vi "CRYHardware Global.vi"() -> ()   [LabVIEW 2013]
panel:
  out "Mic Vol-R backup":dbl
  out "Mic Vol-L backup":dbl
  out "Input Channel 1/2 Index backup":i32
  out "Impedance 1 index backup":i32
  out "Mic Voltage backup":dbl
  out "Mic Res-R backup":dbl
  out "Mic Res-L backup":dbl
  out "Mic Resister backup":dbl
  out "Impedance 2  backup":i32
  out "Impedance 1  backup":i32
  out "Mic Vol-R":dbl
  out "Mic Vol-L":dbl
  out "Input Channel 1/2 Index":i32
  out "Impedance 1 index":i32
  out "Mic Voltage":dbl
  out "Mic Res-R":dbl
  out "Mic Res-L":dbl
  out "Mic Calibration Flag":bool
  out "Mic Resister":dbl
  out "Impedance 2":i32
  out "Impedance 1":i32
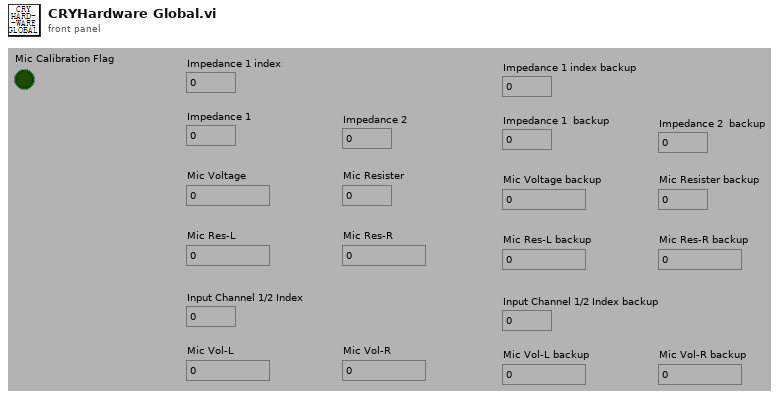
[diagram p1: front panel]
diagram:
